vi "AKIP_query.vi"(8 "error in (no error)":errorcluster, 10 "write buffer":string, 11 "VISA Refnum in":refnum<visa-resource-name>="AKIP") -> (0 "error out":errorcluster, 2 "read buffer":string, 3 "VISA Refnum out":refnum<visa-resource-name>)   [LabVIEW 2017]
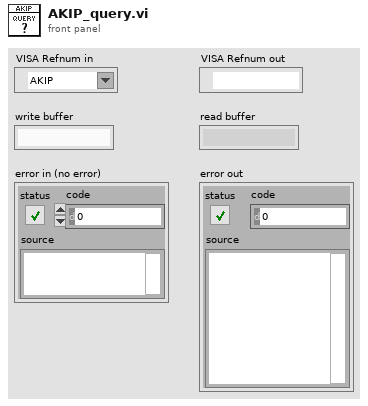
[diagram p1: front panel]
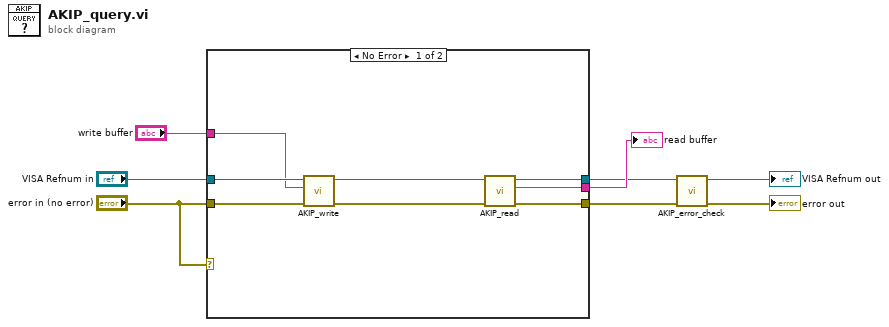
[diagram p0: block diagram]
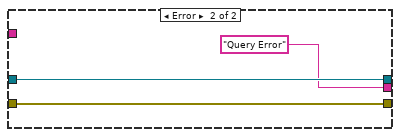
[diagram p2: hidden frame]
diagram:
  n1 = case shown="No Error" "error in (no error)" {
    tunnel: [w16 w19] -> w3
    tunnel: [w15 w18] -> w4
    tunnel: "error in (no error)" -> [w14 w18]
    tunnel: "VISA Refnum in" -> [w13 w19]
    tunnel: [w12 "Query Error" ("read buffer")] -> w7
    tunnel: "write buffer" -> [w11 _]
    frame No Error {
      n2 = call "AKIP_write.vi"("error in (no error)"=w14, "write buffer"=w11, "VISA Refnum in"=w13) -> ("error out"=w9:errorcluster, "VISA Refnum out"=w10:refnum<visa-resource-name>)  [unwired: 7 in]
      n3 = call "AKIP_read.vi"("error in (no error)"=w9, "VISA Refnum in"=w10) -> ("error out"=w15:errorcluster, "read buffer"=w12:string, "VISA Refnum out"=w16:refnum<visa-resource-name>)  [unwired: 7 in]
    }
    frame Error {
    }
  }
  "read buffer" <- w7
  n4 = call "AKIP_error_check.vi"("error in (no error)"=w4, "VISA Refnum in"=w3) -> ("error out"=→"error out":errorcluster, "VISA Refnum out"=→"VISA Refnum out":refnum<visa-resource-name>)  [unwired: 8 in]
